vi "ToArray.vi"(11 "OccupancyGridWorldMap in":refnum<class "NI_Robotics_OccupancyGridWorldMap.lvclass">) -> (2 "cost array":dbl[][](array[numeric]), 3 "OccupancyGridWorldMap out":refnum<class "NI_Robotics_OccupancyGridWorldMap.lvclass">)   [LabVIEW 2017, in "NI_Robotics_OccupancyGridWorldMap.lvclass"]
uses:
  <vilib>/robotics/Navigation/shared/WorldMap/OccupancyGridWorldMap/NI_Robotics_OccupancyGridWorldMap.lvclass
  <vilib>/robotics/Navigation/shared/WorldMap/OccupancyGridWorldMap/NI_Robotics_OccupancyGridWorldMap.lvclass/NI_Robotics_OccupancyGridWorldMap.ctl
  <vilib>/robotics/Navigation/shared/MapNode/OccupancyGridNode/NI_Robotics_OccupancyGridMapNode.lvclass
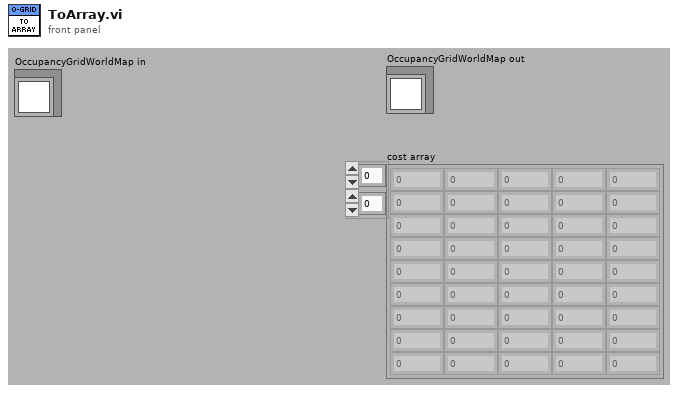
[diagram p1: front panel]
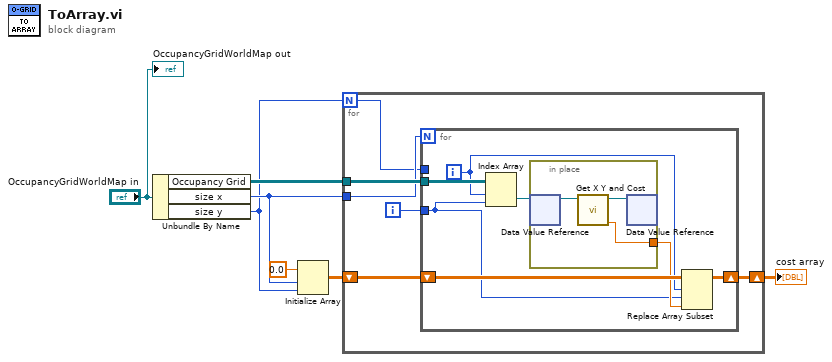
[diagram p0: block diagram]
diagram:
  n1 = Unbundle By Name("OccupancyGridWorldMap in") -> ("Occupancy Grid"=w7:refnum<data-value>[][], "size x"=w5:i32, "size y"=w1:i32)
  n2 = Initialize Array(0.0 ("double precision float"), w5, w1) -> (w6:dbl[][])
  n3 = for {
    N: w1 -> [w10]
    shift-right: [w9] -> w3
    shift-left: w6 -> [w12]
    tunnel: w5 -> [w11]
    tunnel: w7 -> [w13]
    i -> [w8]
    n4 = for {
      N: w11 -> [_]
      shift-right: [w17] -> w9
      shift-left: w12 -> [w19]
      tunnel: w10 -> [_]
      tunnel: w13 -> [w20]
      tunnel: w8 -> [w15]
      i -> [w14]
      n5 = Index Array(array=w20, index (row)=w14, index (col)=w15) -> (element=w18:refnum<data-value>)
      n6 = in-place {
        in-place-border: [w21] -> w16
        n7 = in-place-dvr #1(w18) -> (w23:refnum<class "NI_Robotics_OccupancyGridMapNode.lvclass">)  [unwired: 1 out]
        n8 = call-dynamic "Get X Y and Cost.vi"("OccupancyGridMapNode in"=w23) -> ("Cost"=w21:dbl, "OccupancyGridMapNode out"=w22:refnum<class "NI_Robotics_OccupancyGridMapNode.lvclass">)  [unwired: 7 in, 2 out]
        n9 = in-place-dvr #1(w22) -> ()  [unwired: 2 out]
      }
      n10 = Replace Array Subset(array=w19, new element=w16, index (row)=w14, index (col)=w15) -> (w17:dbl[][])
    }
  }
  "cost array" <- w3
  "OccupancyGridWorldMap out" <- "OccupancyGridWorldMap in"
